vi "Tosca-Read Session Info.vi"(0 "Session Info":T1={"Animal ID"="", "Session"=0, "Path"=path "", "Run"=1} {"Session" min=1 step=1}, 7 "Session Data":string, 11 "error in (no error)":errorcluster) -> (4 "Session Info out":T1={"Animal ID"="", "Session"=0, "Path"=path "", "Run"=1} {"Session" min=1 step=1}, 15 "error out":errorcluster)   [LabVIEW 2020]
uses:
  Typedefs/Tosca-Session Info.ctl
  <vilib>/Utility/config.llb/Read Key (I32).vi
  <vilib>/Utility/config.llb/Write Key (I32).vi
  <vilib>/Utility/config.llb/NI_LVConfig.lvlib
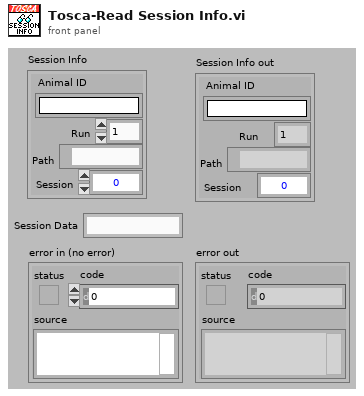
[diagram p1: front panel]
types:
  T1 = typedef "Tosca-Session Info.ctl" = cluster{"Animal ID":string, "Session":i32, "Path":path, "Run":i32}
  T2 = typedef "NI_LVConfig.lvlib/Config Data RefNum.ctl" = refnum<k1>
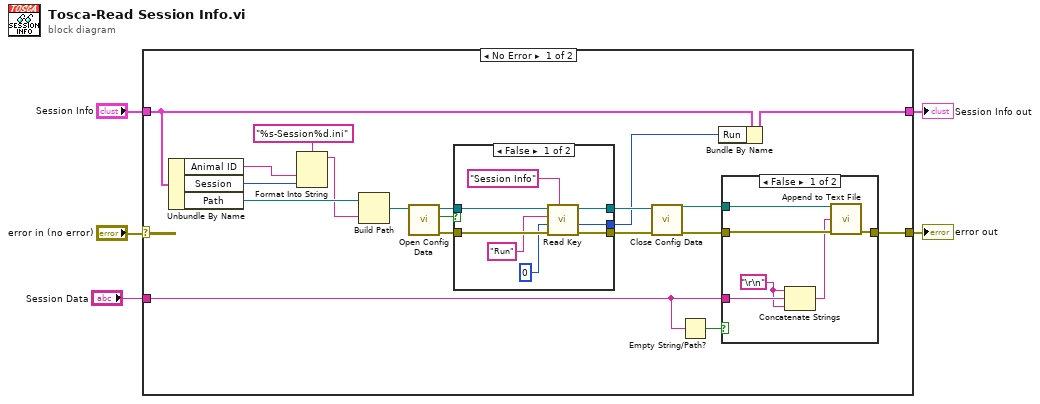
[diagram p0: block diagram]
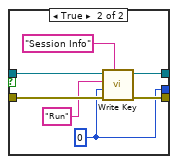
[diagram p2: hidden frame]
diagram:
  n1 = case shown="No Error" "error in (no error)" {
    selector: "error in (no error)" -> [_ w48]
    tunnel: [w10 w48] -> w4
    tunnel: "Session Info" -> [w16 w47]
    tunnel: [w14 w47] -> w2
    tunnel: "Session Data" -> [w8 _]
    frame No Error {
      n2 = Unbundle By Name(w16) -> ("Animal ID"=w12:string, "Session"=w13:i32, "Path"=w23:path)
      n3 = Format Into String(format string="%s-Session%d.ini", w12, w13) -> (resulting string=w22:string)  [unwired: 2 in, 1 out]
      n4 = Build Path(base path=w23, name or relative path=w22) -> (appended path=w21:path)
      n5 = call <vilib>:"Open Config Data.vi"("configuration file path"=w21) -> ("error out"=w20:errorcluster, "file created?"=w6:bool, "refnum"=w19:T2)  [unwired: 8 in]
      n6 = case shown="False" w6 {
        tunnel: w20 -> [w32 w39]
        tunnel: w19 -> [w31 w38]
        tunnel: [w28 w35] -> w18
        tunnel: [w27 w34] -> w17
        tunnel: [w25 w33] -> w15
        frame False {
          n7 = call-poly <vilib>:"Read Key.vi"("section"="Session Info", "error in (no error)"=w32, "default value"=0, "key"="Run", "refnum"=w31) -> ("error out"=w28:errorcluster, "value"=w25:i32, "refnum out"=w27:T2)  [unwired: 3 in, 1 out]
        }
        frame True {
          w33 = 0 ("default value")
          n8 = call-poly <vilib>:"Write Key.vi"("section"="Session Info", "error in (no error)"=w39, "value"=w33, "key"="Run", "refnum"=w38) -> ("error out"=w35:errorcluster, "refnum out"=w34:T2)  [unwired: 4 in, 1 out]
        }
      }
      n9 = call <vilib>:"Close Config Data.vi"("error in (no error)"=w18, "refnum"=w17) -> ("error out"=w9:errorcluster, "file path"=w7:path)  [unwired: 8 in]
      n10 = Empty String/Path?(string/path=w8) -> (empty?=w11:bool)
      n11 = Bundle By Name(cluster=w16, "Run"=w15) -> (w14:T1)
      n12 = case shown="False" w11 {
        tunnel: [w44 w46] -> w10
        tunnel: w9 -> [w45 w46]
        tunnel: w8 -> [w43 _]
        tunnel: w7 -> [w42 _]
        frame False {
          w40 = "\r\n"
          n13 = Concatenate Strings(w40, w43, w40) -> (w41:string)
          n14 = call "Append to Text File.vi"("file path"=w42, "text"=w41, "error in (no error)"=w45) -> ("error out"=w44:errorcluster)  [unwired: 11 in, 1 out]
        }
        frame True {
        }
      }
    }
    frame Error {
    }
  }
  "error out" <- w4
  "Session Info out" <- w2
